vi "Top level wrapper ILD1420.vi"(2 "Reconfigure settings":bool, 3 "ILD1420 COM port":refnum<visa-resource-name>="COM18", 4 "Data rate (kHz)":string(combo)="0.25", 5 "Auto laser off":bool=TRUE, 6 "Measuring range (mm)":u8(ring)=4 items=["10", "25", "50", "100", "200"], 7 "N samples":i32=2000 min=0) -> (0 "Error out":errorcluster, 1 "d (mm)":dbl[](array[numeric]))   [LabVIEW 2020]
uses:
  Globals/ILD1420_Global.vi
  Anemometry/Anemometry Sub Vis/Globals/Meas_global.vi
panel:
  # "(set true if changing data rate)"
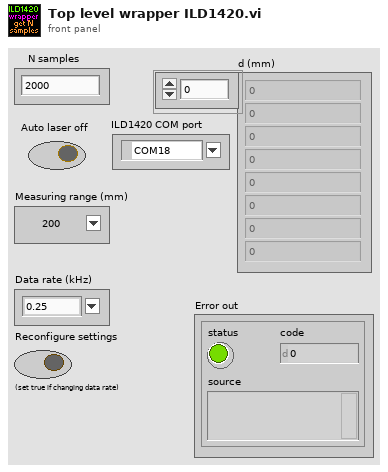
[diagram p1: front panel]
types:
  T1 = typedef "Rendezvous RefNum" = refnum<k1>
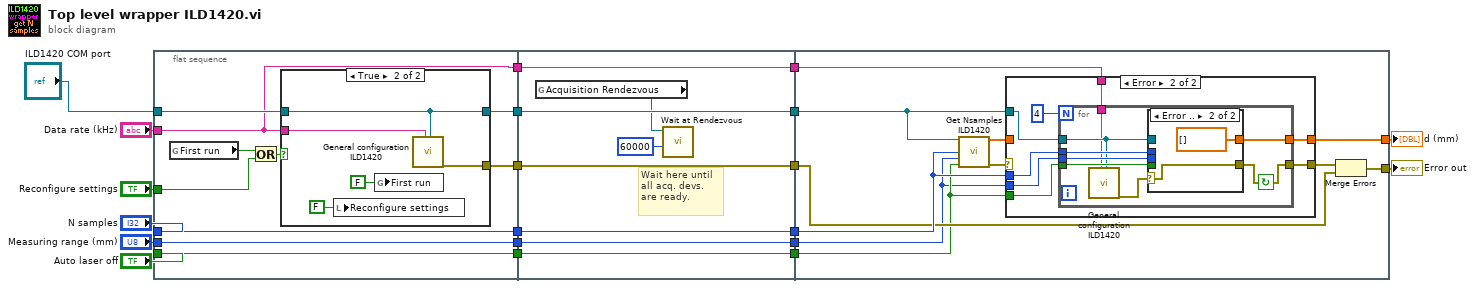
[diagram p0: block diagram]
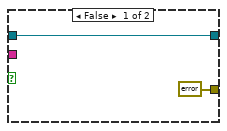
[diagram p2: hidden frame]
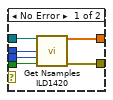
[diagram p4: hidden frame]
diagram:
  n1 = flat-sequence {
    tunnel: "N samples" -> [w30]
    tunnel: [w30] -> w12
    tunnel: [w29] -> w10
    tunnel: [w28] -> w8
    tunnel: "Auto laser off" -> [w28]
    tunnel: [w27] -> w6
    tunnel: "Measuring range (mm)" -> [w27]
    tunnel: "Data rate (kHz)" -> [w21]
    tunnel: "Reconfigure settings" -> [w24]
    tunnel: "ILD1420 COM port" -> [w23]
    tunnel: [w22] -> w4
    tunnel: [w21] -> w2
    tunnel: w12 -> [w45]
    tunnel: [w45] -> w11
    tunnel: w10 -> [w44]
    tunnel: [w44] -> w9
    tunnel: w8 -> [w43]
    tunnel: [w43] -> w7
    tunnel: w6 -> [w42]
    tunnel: [w42] -> w5
    tunnel: w4 -> [w41]
    tunnel: [w41] -> w3
    tunnel: w2 -> [w38]
    tunnel: [w38] -> w1
    tunnel: [w53] -> w20
    tunnel: w11 -> [w54]
    tunnel: [w50] -> w18
    tunnel: w9 -> [w51]
    tunnel: w7 -> [w49]
    tunnel: w5 -> [w48]
    tunnel: w3 -> [w47]
    tunnel: w1 -> [w46]
    frame #0 {
      n2 = global read "ILD1420_Global.vi" "First run"() -> (w25:bool)
      n3 = Or(x=w25, y=w24) -> (x .or. y?=w26:bool)
      n4 = case shown="True" w26 {
        tunnel: [errorcluster {"status"=FALSE, "code"=0, "source"=""} ("Error out") w36] -> w29
        tunnel: w21 -> [_ w35]
        tunnel: w23 -> [w31 w33]
        tunnel: [w31 w33] -> w22
        frame False {
        }
        frame True {
          n5 = local write "Reconfigure settings"(FALSE ("Reconfigure settings")) -> ()
          n6 = global write "ILD1420_Global.vi" "First run"(FALSE ("First run")) -> ()
          n7 = call "General configuration ILD1420.vi"("Data rate (kHz)"=w35, "COM port"=w33) -> ("Error out"=w36:errorcluster)  [unwired: 17 in]
        }
      }
    }
    frame #1 {
      # "Wait here until all acq. devs. are ready."
      n8 = global read "Meas_global.vi" "Acquisition Rendezvous"() -> (w40:T1)
      n9 = call <vilib>:"Wait at Rendezvous.vi"("ms timeout (-1)"=60000, "rendezvous"=w40) -> ()  [unwired: 3 in, 3 out]
    }
    frame #2 {
      n10 = call "Get Nsamples ILD1420.vi"("COM port"=w47, "N samples"=w54, "Measuring range (mm)"=w48, "Auto laser off"=w49) -> ("d (mm)"=w55:dbl[], "Error out"=w56:errorcluster)  [unwired: 10 in]
      n11 = case shown="Error" w56 {
        selector: w56 -> [w57 _]
        tunnel: w55 -> [w58 _]
        tunnel: w54 -> [_ w65]
        tunnel: [w58 w64] -> w53
        tunnel: [w57 w63] -> w52
        tunnel: w49 -> [_ w62]
        tunnel: w48 -> [_ w61]
        tunnel: w47 -> [_ w60]
        tunnel: w46 -> [_ w59]
        frame No Error {
        }
        frame Error {
          n12 = for {
            N: 4 -> [_]
            tunnel: w60 -> [w69]
            tunnel: w65 -> [w74]
            tunnel: [w73] -> w64
            tunnel: [w72] -> w63
            tunnel: w62 -> [w71]
            tunnel: w61 -> [w70]
            tunnel: w59 -> [w68]
            stop <- w72 continue-if-true
            n13 = call "General configuration ILD1420.vi"("Data rate (kHz)"=w68, "COM port"=w69) -> ("Error out"=w67:errorcluster)  [unwired: 17 in]
            n14 = case shown="Error .." w67 {
              selector: w67 -> [_ w81]
              tunnel: w74 -> [w80 _]
              tunnel: [w79 dbl[] [] ("d (mm)")] -> w73
              tunnel: [w78 w81] -> w72
              tunnel: w71 -> [w77 _]
              tunnel: w70 -> [w76 _]
              tunnel: w69 -> [w75 _]
              frame No Error {
                n15 = call "Get Nsamples ILD1420.vi"("COM port"=w75, "N samples"=w80, "Measuring range (mm)"=w76, "Auto laser off"=w77) -> ("d (mm)"=w79:dbl[], "Error out"=w78:errorcluster)  [unwired: 10 in]
              }
              frame Error {
              }
            }
          }
        }
      }
      n16 = Merge Errors(w52, w51) -> (w50:errorcluster)
    }
  }
  "d (mm)" <- w20
  "Error out" <- w18
